vi "Read AO-URLs.vi"(11 "BNT_DAQmx-MCSV in":refnum<class "BNT_DAQmx-MCSV.lvclass">) -> (2 "AO-URLs":string[](array[string]), 3 "BNT_DAQmx-MCSV out":refnum<class "BNT_DAQmx-MCSV.lvclass">)   [LabVIEW 2021, in "BNT_DAQmx.lvlib" / "BNT_DAQmx-MCSV.lvclass"]
uses:
  BNT_DAQmx-MCSV.lvclass
  BNT_DAQmx-MCSV.lvclass/BNT_DAQmx-MCSV.ctl
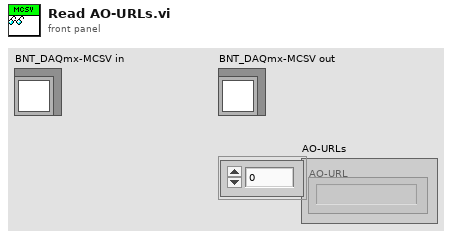
[diagram p1: front panel]
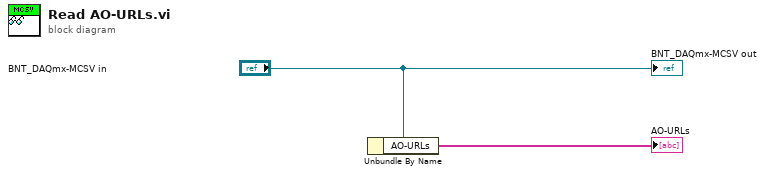
[diagram p0: block diagram]
diagram:
  n1 = Unbundle By Name("BNT_DAQmx-MCSV in") -> ("AO-URLs"=→"AO-URLs":string[])
  "BNT_DAQmx-MCSV out" <- "BNT_DAQmx-MCSV in"
